vi "AD2_linear_sweep_helper.vi"(9 "Freq Sweep (Ch1)":T1, 11 "WFGConfig":T2={"Running"=FALSE, "Ch1"={"idxChannel"=0, "Settings out of range"=FALSE, "Carrier"={"Frequency (Hz)"=0.0, "Amplitude (V)"=1.0, "Offset(V)"=0.0, "Symmetry(%) "=50.0, "Phase(Deg)"=0.0, "Function"=0, "Enable"=FALSE}, "Trigger"={"secRun(0=Cont)"=0.0, "secWait"=0.0, "cRepeat(0=inf)"=0, "Repeat Trigger"=FALSE, "TrigrSrc"=enum."trigrsrcNone"}, "FM Mod"={"Frequency (Hz)"=1000.0, "Amplitude (%)"=1.0, "Offset(V)"=0.0, "Symmetry(%) "=50.0, "Phase(Deg)"=0.0, "Function 2"=1, "Enable"=FALSE}}, "Ch2"={"idxChannel"=1, "Settings out of range"=FALSE, "Carrier"={"Frequency (Hz)"=1000.0, "Amplitude (V)"=1.0, "Offset(V)"=0.0, "Symmetry(%) "=50.0, "Phase(Deg)"=0.0, "Function"=1, "Enable"=FALSE}, "Trigger"={"secRun(0=Cont)"=0.0, "secWait"=0.0, "cRepeat(0=inf)"=0, "Repeat Trigger"=FALSE, "TrigrSrc"=enum."trigrsrcNone"}, "FM Mod"={"Frequency (Hz)"=1000.0, "Amplitude (%)"=1.0, "Offset(V)"=0.0, "Symmetry(%) "=50.0, "Phase(Deg)"=0.0, "Function 2"=1, "Enable"=FALSE}}, "SyncronizeState"=enum."Independent"} {"Ch2"."FM Mod"."Function 2" items=["DC"=0, "Sine"=1, "Square"=2, "Triangle"=3, "RampUp"=4, "RampDown"=5, "Noise"=6, "Pulse"=7, "Custom"=30]; "Ch2"."Carrier"."Function" items=["DC"=0, "Sine"=1, "Square"=2, "Triangle"=3, "RampUp"=4, "RampDown"=5, "Noise"=6, "Pulse"=7, "Custom"=30]; "Ch1"."FM Mod"."Function 2" items=["DC"=0, "Sine"=1, "Square"=2, "Triangle"=3, "RampUp"=4, "RampDown"=5, "Noise"=6, "Pulse"=7, "Custom"=30]; "Ch1"."Carrier"."Function" items=["DC"=0, "Sine"=1, "Square"=2, "Triangle"=3, "RampUp"=4, "RampDown"=5, "Noise"=6, "Pulse"=7, "Custom"=30]}) -> (3 "WFGConfig 2":T2={"Running"=FALSE, "Ch1"={"idxChannel"=0, "Settings out of range"=FALSE, "Carrier"={"Frequency (Hz)"=0.0, "Amplitude (V)"=1.0, "Offset(V)"=0.0, "Symmetry(%) "=50.0, "Phase(Deg)"=0.0, "Function"=0, "Enable"=FALSE}, "Trigger"={"secRun(0=Cont)"=0.0, "secWait"=0.0, "cRepeat(0=inf)"=0, "Repeat Trigger"=FALSE, "TrigrSrc"=enum."trigrsrcNone"}, "FM Mod"={"Frequency (Hz)"=1000.0, "Amplitude (%)"=1.0, "Offset(V)"=0.0, "Symmetry(%) "=50.0, "Phase(Deg)"=0.0, "Function 2"=1, "Enable"=FALSE}}, "Ch2"={"idxChannel"=1, "Settings out of range"=FALSE, "Carrier"={"Frequency (Hz)"=1000.0, "Amplitude (V)"=1.0, "Offset(V)"=0.0, "Symmetry(%) "=50.0, "Phase(Deg)"=0.0, "Function"=1, "Enable"=FALSE}, "Trigger"={"secRun(0=Cont)"=0.0, "secWait"=0.0, "cRepeat(0=inf)"=0, "Repeat Trigger"=FALSE, "TrigrSrc"=enum."trigrsrcNone"}, "FM Mod"={"Frequency (Hz)"=1000.0, "Amplitude (%)"=1.0, "Offset(V)"=0.0, "Symmetry(%) "=50.0, "Phase(Deg)"=0.0, "Function 2"=1, "Enable"=FALSE}}, "SyncronizeState"=enum."Independent"} {"Ch2"."FM Mod"."Function 2" items=["DC"=0, "Sine"=1, "Square"=2, "Triangle"=3, "RampUp"=4, "RampDown"=5, "Noise"=6, "Pulse"=7, "Custom"=30]; "Ch2"."Carrier"."Function" items=["DC"=0, "Sine"=1, "Square"=2, "Triangle"=3, "RampUp"=4, "RampDown"=5, "Noise"=6, "Pulse"=7, "Custom"=30]; "Ch1"."FM Mod"."Function 2" items=["DC"=0, "Sine"=1, "Square"=2, "Triangle"=3, "RampUp"=4, "RampDown"=5, "Noise"=6, "Pulse"=7, "Custom"=30]; "Ch1"."Carrier"."Function" items=["DC"=0, "Sine"=1, "Square"=2, "Triangle"=3, "RampUp"=4, "RampDown"=5, "Noise"=6, "Pulse"=7, "Custom"=30]})   [LabVIEW 2024]
uses:
  AD2_WFG_SDK_class/WFG.ctl
  AD2_WFG_SDK_class/WFGCh.ctl
  AD2_WFG_SDK_class/AD2TriggerSources.ctl
  AD2_SDK_class/AD2_SDK.lvclass
  AD2_WFG_SDK_class/AD2_WFG_SDK.lvclass
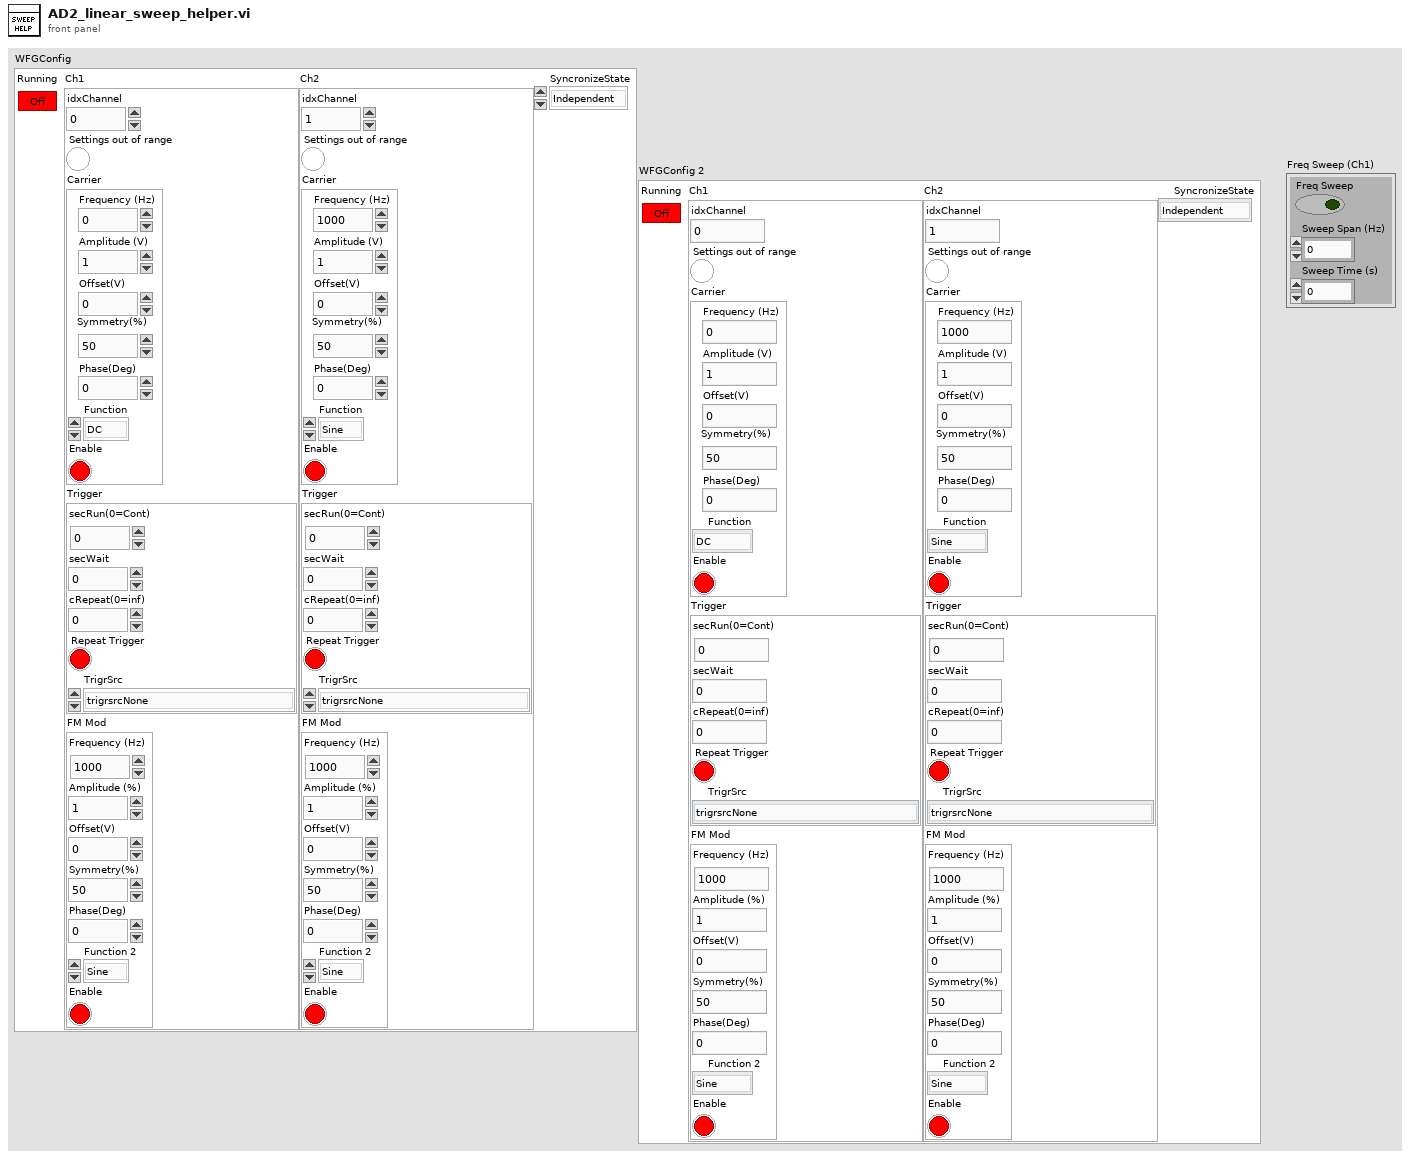
[diagram p1: front panel]
types:
  T1 = cluster{"Freq Sweep":bool, "Sweep Span (Hz)":dbl, "Sweep Time (s)":dbl}
  T2 = typedef "AD2_WFG_SDK.lvclass/WFG.ctl" = cluster{"Running":bool, "Ch1":T3, "Ch2":T3, "SyncronizeState":enum16{"Independent", "Ch1Master", "Ch2Master"}}
  T3 = typedef "AD2_WFG_SDK.lvclass/WFGCh.ctl" = cluster{"idxChannel":i32, "Settings out of range":bool, "Carrier":cluster{"Frequency (Hz)":dbl, "Amplitude (V)":dbl, "Offset(V)":dbl, "Symmetry(%) ":dbl, "Phase(Deg)":dbl, "Function":u16, "Enable":bool}, "Trigger":cluster{"secRun(0=Cont)":dbl, "secWait":dbl, "cRepeat(0=inf)":i32, "Repeat Trigger":bool, "TrigrSrc":T4}, "FM Mod":cluster{"Frequency (Hz)":dbl, "Amplitude (%)":dbl, "Offset(V)":dbl, "Symmetry(%) ":dbl, "Phase(Deg)":dbl, "Function 2":u16, "Enable":bool}}
  T4 = typedef "AD2_SDK.lvclass/AD2TriggerSources.ctl" = enum8{"trigrsrcNone", "trigsrcPC", "trigsrcDetectorAnalogIn", "trigsrcDetectorDigitalIn", "trigsrcAnalogIn", "trigsrcDigitalIn", "trigsrcDigitalOut", "trigsrcAnalogOut1", "trigsrcAnalogOut2", "trigsrcAnalogOut3", "trigsrcAnalogOut4", "trigsrcExternal1", "trigsrcExternal2", "trigsrcExternal3", "trigsrcExternal4", ""}
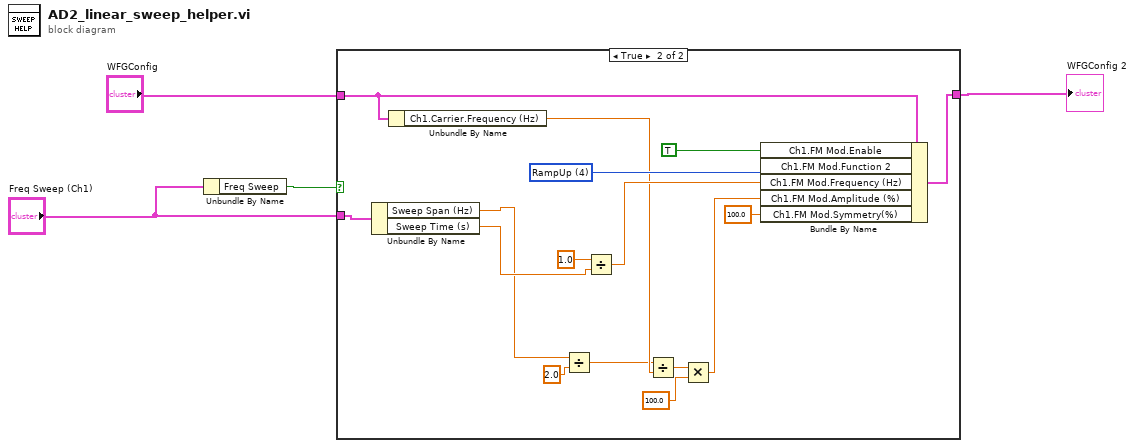
[diagram p0: block diagram]
diagram:
  n1 = Unbundle By Name("Freq Sweep (Ch1)") -> ("Freq Sweep"=w2:bool)
  n2 = case shown="True" w2 {
    tunnel: [w5 w15] -> w4
    tunnel: "WFGConfig" -> [w5 w11]
    tunnel: "Freq Sweep (Ch1)" -> [_ w21]
    frame False {
    }
    frame True {
      w19 = u16 4 items=["DC"=0, "Sine"=1, "Square"=2, "Triangle"=3, "RampUp"=4, "RampDown"=5, "Noise"=6, "Pulse"=7, "Custom"=30] ("Function 2")
      n3 = Unbundle By Name(w21) -> ("Sweep Span (Hz)"=w10:dbl, "Sweep Time (s)"=w17:dbl)
      n4 = Unbundle By Name(w11) -> ("Ch1.Carrier.Frequency (Hz)"=w8:dbl)
      n5 = Divide(x=w10, y=2.0) -> (x/y=w7:dbl)
      n6 = Divide(x=1.0, y=w17) -> (x/y=w16:dbl)
      n7 = Divide(x=w7, y=w8) -> (x/y=w14:dbl)
      n8 = Multiply(x=w14, y=100.0) -> (x*y=w12:dbl)
      n9 = Bundle By Name(cluster=w11, "Ch1.FM Mod.Enable"=TRUE, "Ch1.FM Mod.Function 2"=w19, "Ch1.FM Mod.Frequency (Hz)"=w16, "Ch1.FM Mod.Amplitude (%)"=w12, "Ch1.FM Mod.Symmetry(%)"=100.0) -> (w15:T2)
    }
  }
  "WFGConfig 2" <- w4
